vi "Construct.vi"(8 "error in (no error)":errorcluster, 9 "VI Path (Relative)":path, 10 "Resource Data ref":refnum<data-value>, 11 "LVProject File Path (Absolute)":path) -> (0 "error out":errorcluster, 3 "VI Data out":refnum<class "VI Data.lvclass">)   [LabVIEW 2013, in "SET Project Data.lvlib" / "VI Data.lvclass"]
uses:
  VI Data.lvclass
  Resource Data Class/Resource Data.lvclass
  VI Data.lvclass/VI Data.ctl
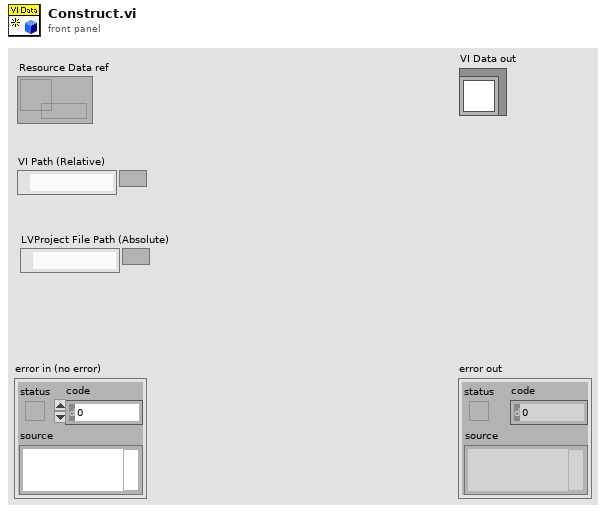
[diagram p1: front panel]
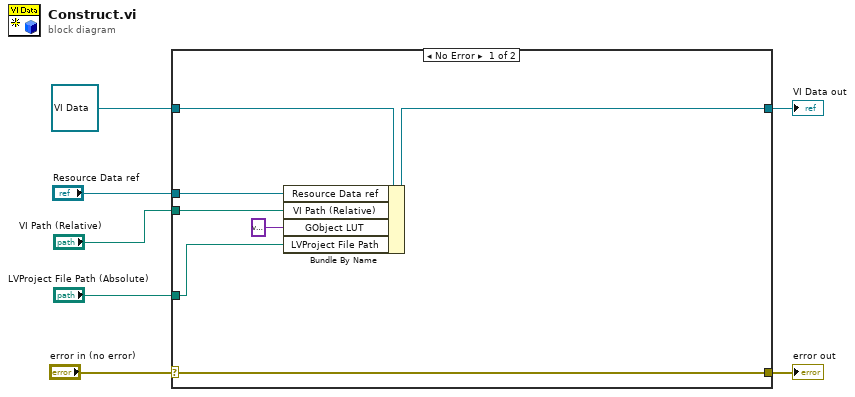
[diagram p0: block diagram]
diagram:
  n1 = case shown="No Error" "error in (no error)" {
    selector: "error in (no error)" -> [w14 w16]
    tunnel: [w14 w16] -> w6
    tunnel: [w12 w15] -> w5
    tunnel: refnum<class "VI Data.lvclass"> refnum ("SET VI in") -> [w13 w15]
    tunnel: "Resource Data ref" -> [w11 _]
    tunnel: "VI Path (Relative)" -> [w10 _]
    tunnel: "LVProject File Path (Absolute)" -> [w8 _]
    frame No Error {
      n2 = Bundle By Name(cluster=w13, "Resource Data ref"=w11, "VI Path (Relative)"=w10, "GObject LUT"=variant, "LVProject File Path"=w8) -> (w12:refnum<class "VI Data.lvclass">)
    }
    frame Error {
    }
  }
  "error out" <- w6
  "VI Data out" <- w5
